vi "update Neurophotometrics FP3002.vi"() -> ()   [LabVIEW 2010]
panel:
  in  "Update":bool
  in  "Firmware file for Screen":path
  in  "VISA resource name":refnum<visa-resource-name>
  in  "Firmware file for Master":path
  # "v1.0"
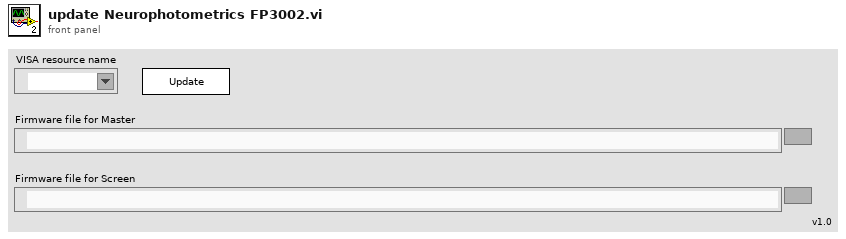
[diagram p1: front panel]
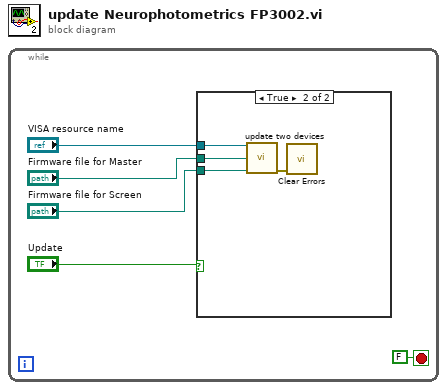
[diagram p0: block diagram]
diagram:
  n1 = while {
    stop <- FALSE ("stop") stop-if-true
    n2 = case shown="True" "Update" {
      tunnel: "VISA resource name" -> [_ w9]
      tunnel: "Firmware file for Master" -> [_ w8]
      tunnel: "Firmware file for Screen" -> [_ w7]
      frame False {
      }
      frame True {
        n3 = call "update two devices.vi"("VISA resource name"=w9, "Firmware file for Master"=w8, "Firmware file for Screen"=w7) -> ("error out"=w6:errorcluster)  [unwired: 12 in]
        n4 = call <vilib>:"Clear Errors.vi"("error in (no error)"=w6) -> ()  [unwired: 6 in, 1 out]
      }
    }
  }
